vi "testGetViGetNextSample.vi"(8 "error in (no error)":errorcluster) -> (0 "error out":errorcluster)   [LabVIEW 2018]
uses:
  src/LibReader/LibReader.lvclass
  <vilib>/addons/_JKI Toolkits/Caraya/classes/Assert/Assert Equal Value_Variant.vi
  <vilib>/addons/_JKI Toolkits/Caraya/classes/Assert/Assert Error.vi
  <vilib>/addons/_JKI Toolkits/Caraya/classes/Test/Test.lvclass
  <vilib>/addons/_JKI Toolkits/Caraya/classes/Assert/Assert.lvclass
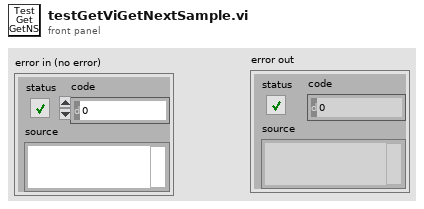
[diagram p1: front panel]
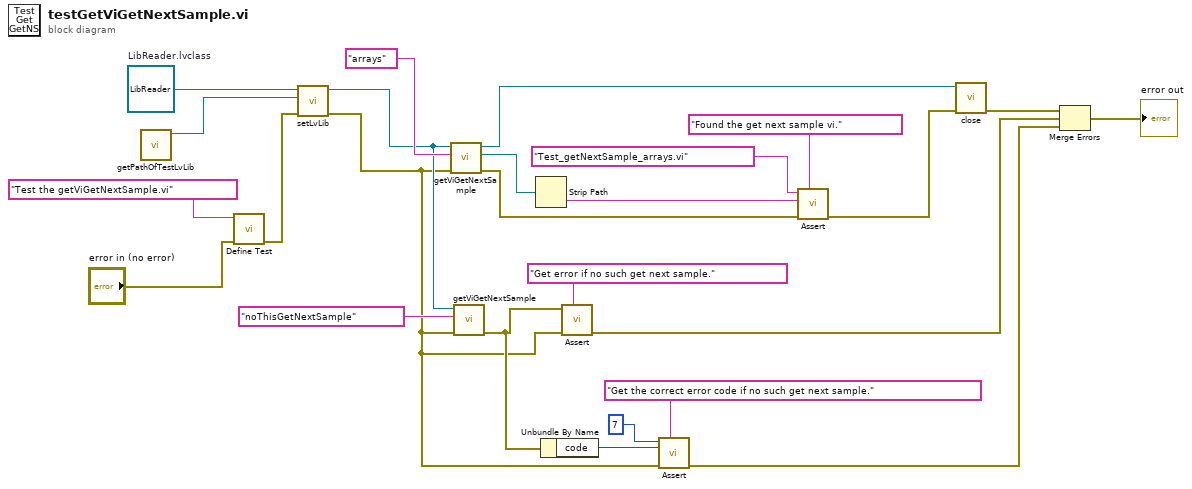
[diagram p0: block diagram]
diagram:
  w23 = refnum<class "LibReader.lvclass"> refnum  # LibReader.lvclass
  n1 = call "getPathOfTestLvLib.vi"() -> ("testLvLibPath"=w22:path)  [unwired: 11 in]
  n2 = call <vilib>:"Define Test.vi"("error in (no error)"="error in (no error)", "Label (VI Title)"="Test the getViGetNextSample.vi") -> ("error out"=w21:errorcluster)  [unwired: 9 in]
  n3 = call "setLvLib.vi"("error in (no error)"=w21, "pathLvLib"=w22, "LibReader in"=w23) -> ("error out"=w1:errorcluster, "LibReader out"=w12:refnum<class "LibReader.lvclass">)  [unwired: 7 in]
  n4 = call "getViGetNextSample.vi"("error in (no error)"=w1, "name"="arrays", "LibReader in"=w12) -> ("error out"=w17:errorcluster, "pathViGetNextSample"=w19:path, "LibReader out"=w20:refnum<class "LibReader.lvclass">)  [unwired: 6 in]
  n5 = call "getViGetNextSample.vi"("error in (no error)"=w1, "name"="noThisGetNextSample", "LibReader in"=w12) -> ("error out"=w3:errorcluster)  [unwired: 6 in, 2 out]
  n6 = Strip Path(path=w19) -> (name=w18:string)  [unwired: 1 out]
  n7 = Unbundle By Name(w3) -> ("code"=w6:i32)
  n8 = call-poly <vilib>:"Assert.vi"("Label"="Get error if no such get next sample.", "error in (no error)"=w1, "Error?"=w3) -> ("error out"=w7:errorcluster)  [unwired: 8 in]
  n9 = call-poly <vilib>:"Assert.vi"("Label"="Get the correct error code if no such get next sample.", "error in (no error)"=w1, "Y"=w6, "X"=7) -> ("error out"=w2:errorcluster)  [unwired: 7 in]
  n10 = call-poly <vilib>:"Assert.vi"("Label"="Found the get next sample vi.", "error in (no error)"=w17, "Y"=w18, "X"="Test_getNextSample_arrays.vi") -> ("error out"=w16:errorcluster)  [unwired: 7 in]
  n11 = call "close.vi"("error in (no error)"=w16, "LibReader in"=w20) -> ("error out"=w9:errorcluster)  [unwired: 8 in, 1 out]
  n12 = Merge Errors(w9, w7, w2) -> (→"error out":errorcluster)
